vi "Set Acquisition Config.vi"(8 "error in (no error)":errorcluster, 10 "Cluster":T1={"signal type"=enum."Sine Wave", "sampling info"={"Fs"=1000.0, "#s"=1000.0}, "frequency"=10.0, "amplitude"=1.0, "square wave duty cycle (%)"=50.0, "offset"=0.0, "phase"=0.0}) -> (0 "error out":errorcluster)   [LabVIEW 2020, in "Acquisiton Oscar Template.lvlib"]
doc: "Set the wavwfrm parameters for acquisition\n_____\nCreated using Delacor QMH Event Scripter 5.0.0.112."
uses:
  Acquisiton Oscar Template.lvlib
  Set Acquisition Config Argument--cluster.ctl
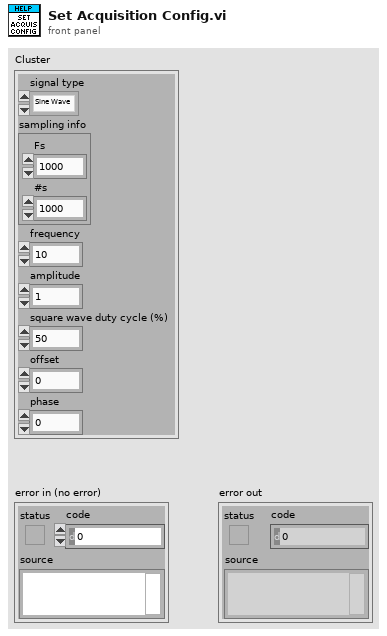
[diagram p1: front panel]
types:
  T1 = cluster{"signal type":enum16{"Sine Wave", "Triangle Wave", "Square Wave", "Sawtooth Wave"}, "sampling info":cluster{"Fs":dbl, "#s":dbl}, "frequency":dbl, "amplitude":dbl, "square wave duty cycle (%)":dbl, "offset":dbl, "phase":dbl}
  T2 = typedef "Acquisiton Oscar Template.lvlib/Set Acquisition Config Argument--cluster.ctl" = cluster{"Cluster":cluster{"signal type":enum16{"Sine Wave", "Triangle Wave", "Square Wave", "Sawtooth Wave"}, "sampling info":cluster{"Fs":dbl, "#s":dbl}, "frequency":dbl, "amplitude":dbl, "square wave duty cycle (%)":dbl, "offset":dbl, "phase":dbl}}
  T3 = typedef "Acquisiton Oscar Template.lvlib/Request Events--cluster.ctl" = cluster{"Stop Module":refnum<user-event>, "Show Panel":refnum<user-event>, "Hide Panel":refnum<user-event>, "Get Module Execution Status":refnum<user-event>, "Show Diagram":refnum<user-event>, "Start Helper Loop":refnum<user-event>, "Stop Helper Loop":refnum<user-event>, "Set Acquisition Config":refnum<user-event>}
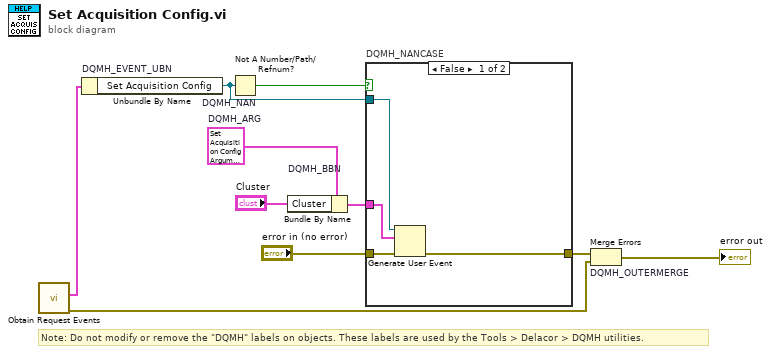
[diagram p0: block diagram]
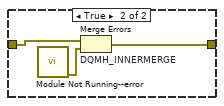
[diagram p2: hidden frame]
diagram:
  w4 = T2 {"Cluster"={"signal type"=enum."Sine Wave", "sampling info"={"Fs"=1000.0, "#s"=1000.0}, "frequency"=10.0, "amplitude"=1.0, "square wave duty cycle (%)"=50.0, "offset"=0.0, "phase"=0.0}}  # DQMH_ARG
  # "Note: Do not modify or remove the \"DQMH\" labels on objects. These labels are used by the Tools > Delacor > DQMH utilities."
  n1 = call "Obtain Request Events.vi"() -> ("error out"=w2:errorcluster, "Acquisiton Oscar Template Request Events"=w1:T3)  [unwired: 10 in]
  n2 = Unbundle By Name "DQMH_EVENT_UBN"(w1) -> ("Set Acquisition Config"=w6:refnum<user-event>)
  n3 = Not A Number/Path/Refnum? "DQMH_NAN"(number/path/refnum=w6) -> (NaN/Path/Refnum?=w7:bool)
  n4 = Bundle By Name "DQMH_BBN"(cluster=w4, "Cluster"="Cluster") -> (w8:T2)
  n5 = case "DQMH_NANCASE" shown="False" w7 {
    tunnel: "error in (no error)" -> [w14 w17]
    tunnel: [w13 w16] -> w5
    tunnel: w6 -> [w12 _]
    tunnel: w8 -> [w11 _]
    frame False {
      n6 = Generate User Event(user event=w12, event data cluster=w11, error in=w14) -> (error out=w13:errorcluster)  [unwired: 1 in, 1 out]
    }
    frame True {
      n7 = call "Module Not Running--error.vi"() -> ("error out"=w15:errorcluster)  [unwired: 11 in]
      n8 = Merge Errors "DQMH_INNERMERGE"(w17, w15) -> (w16:errorcluster)
    }
  }
  n9 = Merge Errors "DQMH_OUTERMERGE"(w5, w2) -> (→"error out":errorcluster)
